vi "abs.vi"(10 "Boolean 2":bool, 11 "PWM_in":dbl) -> (3 "PWM_out":dbl)   [LabVIEW 2016]
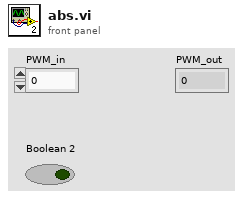
[diagram p1: front panel]
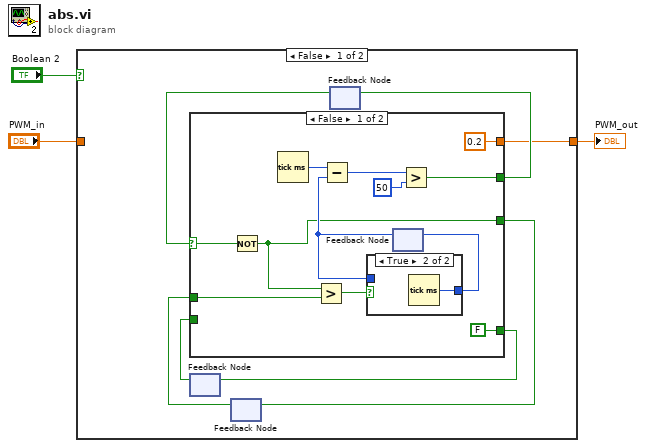
[diagram p0: block diagram]
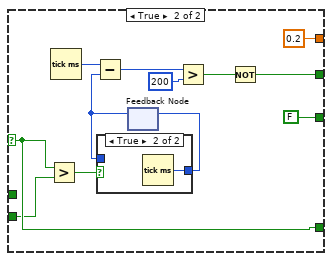
[diagram p3: hidden frame]
diagram:
  n1 = case shown="False" "Boolean 2" {
    tunnel: "PWM_in" -> [_ w39]
    tunnel: [w8 w39] -> w2
    frame False {
      n2 = feedback #1() -> (w4:bool)  [unwired: 1 in]
      n3 = feedback #2() -> (w6:bool)  [unwired: 1 in]
      n4 = feedback #3() -> (w9:bool)  [unwired: 1 in]
      n5 = case shown="False" w9 {
        selector: w9 -> [w15 w26]
        tunnel: [w16 w29] -> w10
        tunnel: [0.2 0.2] -> w8
        tunnel: [w13 FALSE] -> w7
        tunnel: w6 -> [w12 _]
        tunnel: [FALSE w26] -> w5
        tunnel: w4 -> [_ w25]
        frame False {
          n6 = Not(x=w15) -> (.not. x?=w13:bool)
          n7 = Tick Count (ms)() -> (millisecond timer value=w19:u32)
          n8 = Greater?(x=w13, y=w12) -> (0:w17:bool)
          n9 = feedback #4() -> (w20:u32)  [unwired: 1 in]
          n10 = Subtract(x=w19, y=w20) -> (x-y=w21:u32)
          n11 = case shown="True" w17 {
            tunnel: w20 -> [w23 _]
            tunnel: [w23 w24] -> w18
            frame False {
            }
            frame True {
              n12 = Tick Count (ms)() -> (millisecond timer value=w24:u32)
            }
          }
          n13 = feedback-in #4(w18) -> ()
          n14 = Greater?(x=w21, y=u32 50) -> (0:w16:bool)
        }
        frame True {
          n15 = Greater?(x=w26, y=w25) -> (0:w36:bool)
          n16 = Tick Count (ms)() -> (millisecond timer value=w34:u32)
          n17 = feedback #5() -> (w33:u32)  [unwired: 1 in]
          n18 = Subtract(x=w34, y=w33) -> (x-y=w32:u32)
          n19 = case shown="True" w36 {
            tunnel: w33 -> [w37 _]
            tunnel: [w37 w38] -> w35
            frame False {
            }
            frame True {
              n20 = Tick Count (ms)() -> (millisecond timer value=w38:u32)
            }
          }
          n21 = feedback-in #5(w35) -> ()
          n22 = Greater?(x=w32, y=u32 200) -> (0:w30:bool)
          n23 = Not(x=w30) -> (.not. x?=w29:bool)
        }
      }
      n24 = feedback-in #1(w5) -> ()
      n25 = feedback-in #2(w7) -> ()
      n26 = feedback-in #3(w10) -> ()
    }
    frame True {
    }
  }
  "PWM_out" <- w2
